vi "Test Node Guarding.vi"(11 "Test Case In":refnum<class "Tests Network Manager.lvclass">) -> (0 "error out":errorcluster, 3 "Test Case Out":refnum<class "Tests Network Manager.lvclass">)   [LabVIEW 2020, in "Tests Network Manager.lvclass"]
uses:
  <vilib>/Astemes/LUnit/Test Case.lvclass/Test Case.ctl
  Tests Network Manager.lvclass
  Tests Network Manager.lvclass/Tests Network Manager.ctl
  HAL/Source/Communicator/Communicator.lvclass
  D:/git/HAL/Source/Interfaces/IInstrument/IInstrument.lvclass
  D:/git/HAL/Source/Interfaces/IClose/IClose.lvclass
  D:/git/HAL/Source/Interfaces/IInitialize/IInitialize.lvclass
  D:/git/HAL/Source/Communicator/Communicator.lvclass
  D:/git/HAL/Source/Interfaces/ICommunicate/ICommunicate.lvclass
  D:/git/HAL/Source/Interfaces/IConfigurable/IConfigurable.lvclass
  D:/git/HAL/Source/Interfaces/IRunnable/IRunnable.lvclass
  HAL/HAL-Devices/source/PCAN USB Dongle/PCAN Basic 4/Configure Strategies/Read-Write CAN Frame Strategy/PCAN Basic4 Read-Write CAN CC Frame Strategy.lvclass
  D:/git/HAL/HAL-Devices/source/PCAN USB Dongle/PCAN Basic 4/Configure Strategies/Base Configure Strategy/PCAN Basic4 Base Configure Strategy.lvclass
  D:/git/HAL/Source/Interfaces/IApplyConfiguration/IApplyConfiguration.lvclass
  D:/git/HAL/Source/Interfaces/IValidate Configuration/IValidate Configuration.lvclass
  D:/git/HAL/HAL-Devices/source/PCAN USB Dongle/PCAN Basic 4/Configure Strategies/Read-Write CAN Frame Strategy/PCAN Basic4 Read-Write CAN CC Frame Strategy.lvclass
  source/Logging/Logger/Logger.lvclass
  C:/Program Files/National Instruments/LabVIEW 2026/vi.lib/ActorFramework/Actor/Actor.lvclass
  D:/git/CANopen-LabVIEW/source/Logging/Logger/Logger.lvclass
  4993e8ee-a06a-463a-9684-69129f64d5ce.vi
  source/Logging/Log Level.vi
  source/Logging/CANopen Logging.lvlib
  <vilib>/ActorFramework/Actor/Actor.lvclass
  <vilib>/ActorFramework/Stop Msg/Stop Msg.lvclass
  source/SDO Manager/SDO Manager/SDO Manager/SDO Manager.lvclass
  source/Typedefs/Multiplexer.ctl
  source/CANopen.lvlib
  source/SDO Manager/SDO Manager/SDO Manager/Download U16.vi
  source/SDO Manager/SDO Manager/SDO Manager/Download U8.vi
  source/Network Management/Network Management/Network Management.lvclass
panel:
  out "State":u16
  out "Node ID":u8
  out "Octet String":string
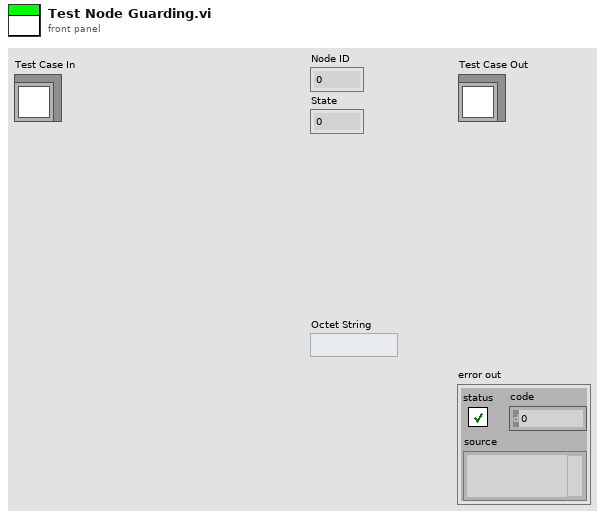
[diagram p1: front panel]
types:
  T1 = cluster{"Guard time (ms)":i32, "Lifetime Factor":u8}
  T2 = typedef "CANopen.lvlib/Multiplexer.ctl" = cluster{"Index":u16, "Sub Index":u8}
  T3 = enum16{"Error", "Warn", "Info", "Debug", "Trace"}
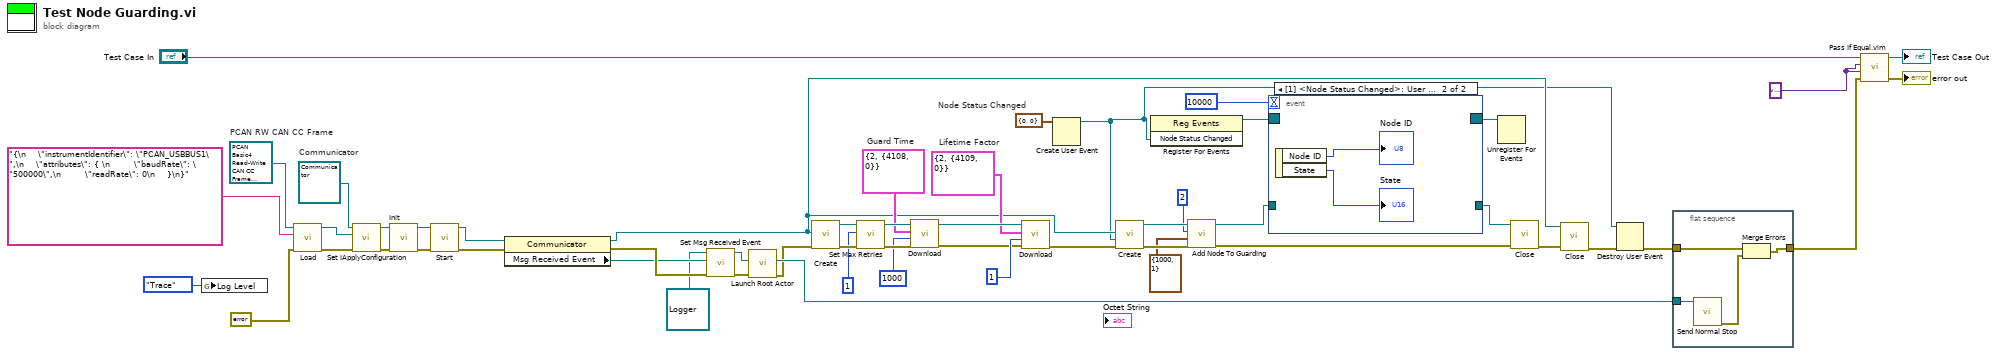
[diagram p0: block diagram]
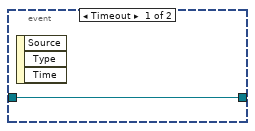
[diagram p2: hidden frame]
diagram:
  w3 = variant ("Expected")
  w19 = cluster{"Node-ID":u8, "Multiplexer":T2} {"Node-ID"=2, "Multiplexer"={"Index"=4109, "Sub Index"=0}}  # Lifetime Factor
  w22 = cluster{"Node-ID":u8, "Multiplexer":T2} {"Node-ID"=2, "Multiplexer"={"Index"=4108, "Sub Index"=0}}  # Guard Time
  w30 = cluster{"Node ID":u8, "State":u16} {"Node ID"=0, "State"=0}  # Node Status Changed
  w38 = refnum<class "Communicator.lvclass"> refnum  # Communicator
  w43 = refnum<class "PCAN Basic4 Read-Write CAN CC Frame Strategy.lvclass"> refnum  # PCAN RW CAN CC Frame
  n1 = global write "Log Level.vi" "Log Level"(T3."Trace" ("Log Level")) -> ()
  n2 = call-dynamic "Load.vi"("error in"=errorcluster {"status"=FALSE, "code"=0, "source"=""} ("error constant"), "Source"="{\n    \"instrumentIdentifier\": \"PCAN_USBBUS1\",\n    \"attributes\": { \n        \"baudRate\": \"500000\",\n        \"readRate\": 0\n    }\n}", "PCAN Basic Base Configure Strategy in"=w43) -> ("error out"=w41:errorcluster, "PCAN Basic Base Configure Strategy out"=w42:refnum<class "PCAN Basic4 Read-Write CAN CC Frame Strategy.lvclass">)  [unwired: 7 in]
  n3 = call-dynamic "Set IApplyConfiguration.vi"("Error In"=w41, "IApplyConfiguration"=w42, "Communicator in"=w38) -> ("Error Out"=w40:errorcluster, "Communicator out"=w39:refnum<class "Communicator.lvclass">)  [unwired: 7 in]
  n4 = call-dynamic "Init.vi"("Error In"=w40, "Communicator in"=w39) -> ("Error Out"=w37:errorcluster, "Communicator out"=w36:refnum<class "Communicator.lvclass">)  [unwired: 8 in]
  n5 = call-dynamic "Start.vi"("Error In"=w37, "Communicator in"=w36) -> ("Error Out"=w35:errorcluster, "Communicator out"=w34:refnum<class "Communicator.lvclass">)  [unwired: 8 in]
  n6 = property class="Communicator"(reference=w34, error in=w35) -> (reference out=w8:refnum<class "Communicator.lvclass">, error out=w48:errorcluster, "Msg Received Event"=w47:refnum<user-event>)
  n7 = call "Set Msg Received Event.vi"("error in"=w48, "Msg Received Event"=w47, "Logger in"=refnum<class "Logger.lvclass"> refnum) -> ("error out"=w50:errorcluster, "Logger out"=w49:refnum<class "Logger.lvclass">)  [unwired: 7 in]
  n8 = call <vilib>:"Launch Root Actor.vi"("error in (no error)"=w50, "Actor"=w49) -> ("error out"=w31:errorcluster, "Actor's Enqueuer"=w44:refnum<class "Message Enqueuer.lvclass">)  [unwired: 8 in]
  n9 = call "Create.vi"("Error In"=w31, "ICommunicate"=w8) -> ("Error Out"=w27:errorcluster, "SDO Manager"=w26:refnum<class "SDO Manager.lvclass">)  [unwired: 8 in]
  n10 = call "Set Max Retries.vi"("error in"=w27, "Max Retries"=u8 1, "SDO Manager in"=w26) -> ("error out"=w24:errorcluster, "SDO Manager out"=w23:refnum<class "SDO Manager.lvclass">)  [unwired: 7 in]
  n11 = call-poly "Download.vi"("error in"=w24, "Value"=u16 1000, "Parameters"=w22, "SDO Manager in"=w23) -> ("error out"=w13:errorcluster, "SDO Manager out"=w20:refnum<class "SDO Manager.lvclass">)  [unwired: 5 in, 1 out]
  n12 = call-poly "Download.vi"("error in"=w13, "Value"=u8 1, "Parameters"=w19, "SDO Manager in"=w20) -> ("error out"=w12:errorcluster)  [unwired: 5 in, 2 out]
  n13 = Create User Event(user event datatype=w30) -> (user event=w5:refnum<user-event>)  [unwired: 1 in, 1 out]
  n14 = call "Create.vi"("error in"=w12, "Node Status Changed"=w5, "ICommunicate"=w8) -> ("error out"=w18:errorcluster, "Network Management"=w17:refnum<class "Network Management.lvclass">)  [unwired: 7 in]
  n15 = register-events(w5) -> (reference out=w4:refnum<event-registration>)  [unwired: 2 in, 1 out]
  n16 = call "Add Node To Guarding.vi"("error in"=w18, "Timings"=T1 {"Guard time (ms)"=1000, "Lifetime Factor"=1}, "Node ID"=u8 2, "Network Management in"=w17) -> ("error out"=w10:errorcluster, "Network Management out"=w1:refnum<class "Network Management.lvclass">)  [unwired: 6 in]
  n17 = event shown="[1] <Node Status Changed>: User Event" {
    selector: w4 -> [_ _]
    dyn-events: [_ _] -> w6
    timeout: 10000 -> [_ _]
    tunnel: [w54 _] -> w2
    tunnel: w1 -> [w54 _]
    event Timeout {
      n18 = event-data() -> ()  [unwired: 1 in, 3 out]
    }
    event User Event {
      n19 = event-data() -> ("Node ID"=→"Node ID":u8, "State"=→"State":u16)  [unwired: 1 in]
    }
  }
  n20 = Unregister For Events(event registration refnum=w6) -> ()  [unwired: 1 in, 1 out]
  n21 = call "Close.vi"("error in"=w10, "Network Management in"=w2) -> ("error out"=w9:errorcluster)  [unwired: 8 in, 1 out]
  n22 = call-dynamic "Close.vi"("Error In"=w9, "Communicator in"=w8) -> ("Error Out"=w45:errorcluster)  [unwired: 8 in, 1 out]
  n23 = Destroy User Event(user event=w5, error in=w45) -> (error out=w7:errorcluster)
  n24 = flat-sequence {
    tunnel: w7 -> [w57]
    tunnel: w44 -> [w60]
    tunnel: [w58] -> w32
    frame #0 {
      n25 = call <vilib>:"Send Normal Stop.vi"("Message Enqueuer"=w60) -> ("error out"=w59:errorcluster)  [unwired: 10 in]
      n26 = Merge Errors(w57, w59) -> (w58:errorcluster)
    }
  }
  n27 = call "Pass If Equal.vim"("error in (no error)"=w32, "Actual"=w3, "Expected"=w3, "LUnit Test Case In"="Test Case In") -> ("error out"=→"error out":errorcluster, "LUnit Test Case Out"=→"Test Case Out":refnum<class "Tests Network Manager.lvclass">)  [unwired: 6 in]
